vi "MakeExample.vi"(8 "error in (no error)":errorcluster, 9 "TriggerRefractoryPeriod (Frames)":i32, 10 "StimulusObject Parameters":variant, 11 "FullWormGWN in":refnum<class "FullWormGWN.lvclass">) -> (0 "error out":errorcluster, 3 "FullWormGWN out":refnum<class "FullWormGWN.lvclass">)   [LabVIEW 2019, in "FullWormGWN.lvclass"]
uses:
  FullWormGWN.lvclass
  FullWormGWNInputCluster.ctl
  FullWormGWN.lvclass/FullWormGWN.ctl
  ParametersGlobal.vi
  StimulusObject.lvclass
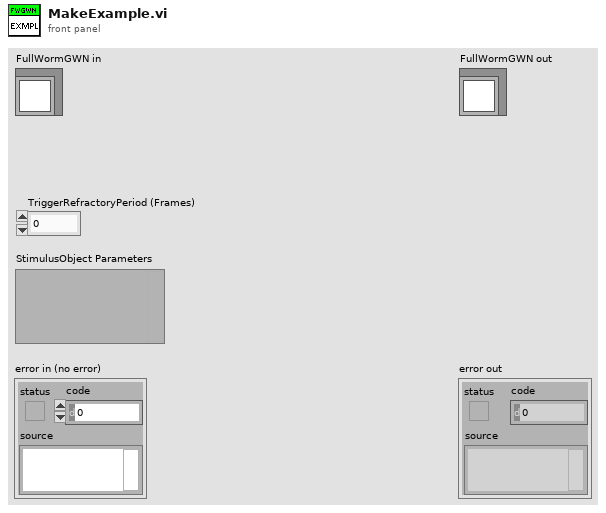
[diagram p1: front panel]
types:
  T1 = typedef "FullWormGWN.lvclass/FullWormGWNInputCluster.ctl" = cluster{"offset (red uW/mm^2m, blue is negative)":sgl, "correlation time (s)":sgl, "standard deviation (red uW/mm^2)":sgl, "Max blue stimulus (uW/mm^2)":sgl, "Max red stimulus (uW/mm^2)":sgl, "dot radius (mm)":sgl}
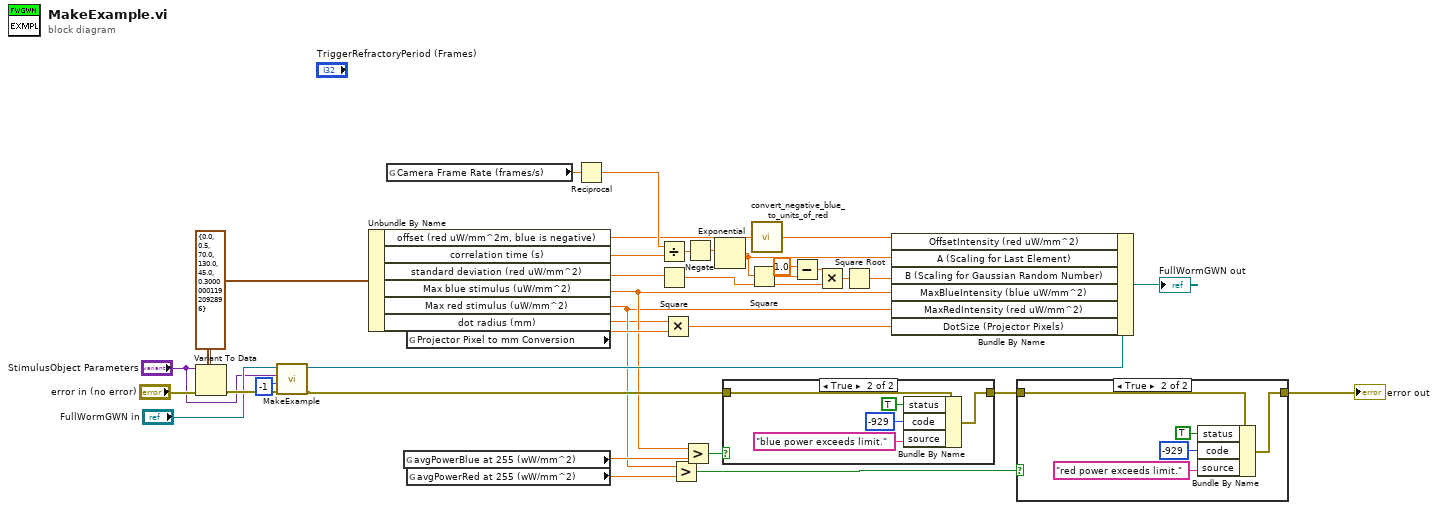
[diagram p0: block diagram]
diagram:
  n1 = Variant To Data(error in="error in (no error)", type=T1 {"offset (red uW/mm^2m, blue is negative)"=0.0, "correlation time (s)"=0.5, "standard deviation (red uW/mm^2)"=70.0, "Max blue stimulus (uW/mm^2)"=130.0, "Max red stimulus (uW/mm^2)"=45.0, "dot radius (mm)"=0.3} ("FullWormGWNInputCluster"), Variant="StimulusObject Parameters") -> (data=w15:T1, error out=w14:errorcluster)
  n2 = call-parent "MakeExample.vi"("error in (no error)"=w14, "TriggerRefractoryPeriod (Frames)"=-1, "StimulusObject Parameters"="StimulusObject Parameters", "StimulusObject in"="FullWormGWN in") -> ("error out"=w20:errorcluster, "StimulusObject out"=w36:refnum<class "FullWormGWN.lvclass">)  [unwired: 6 in]
  n3 = Unbundle By Name(w15) -> ("offset (red uW/mm^2m, blue is negative)"=w7:sgl, "correlation time (s)"=w13:sgl, "standard deviation (red uW/mm^2)"=w12:sgl, "Max blue stimulus (uW/mm^2)"=w11:sgl, "Max red stimulus (uW/mm^2)"=w10:sgl, "dot radius (mm)"=w9:sgl)
  n4 = global read "ParametersGlobal.vi" "Camera Frame Rate (frames/s)"() -> (w27:sgl)
  n5 = global read "ParametersGlobal.vi" "avgPowerBlue at 255 (wW/mm^2)"() -> (w22:sgl)
  n6 = global read "ParametersGlobal.vi" "Projector Pixel to mm Conversion"() -> (w26:sgl)
  n7 = global read "ParametersGlobal.vi" "avgPowerRed at 255 (wW/mm^2)"() -> (w21:sgl)
  n8 = Reciprocal(x=w27) -> (1/x=w29:sgl)
  n9 = Divide(x=w29, y=w13) -> (x/y=w30:sgl)
  n10 = Square(x=w12) -> (x^2=w34:sgl)
  n11 = Multiply(x=w9, y=w26) -> (x*y=w25:sgl)
  n12 = Greater?(x=w10, y=w21) -> (0:w17:bool)
  n13 = Greater?(x=w11, y=w22) -> (0:w19:bool)
  n14 = Negate(x=w30) -> (-x=w31:sgl)
  n15 = Exponential(1:w31) -> (0:w24:sgl)
  n16 = case shown="True" w19 {
    tunnel: w20 -> [w37 w42]
    tunnel: [w37 w41] -> w18
    frame False {
    }
    frame True {
      n17 = Bundle By Name(cluster=w42, "status"=TRUE, "code"=-929, "source"="blue power exceeds limit.") -> (w41:errorcluster)
    }
  }
  n18 = Square(x=w24) -> (x^2=w32:sgl)
  n19 = call "convert_negative_blue_to_units_of_red.vi"("Intensity in units of red (positive) and blue (negative)"=w7) -> ("Intensity in units of red (positive and negative)"=w6:sgl)
  n20 = Subtract(x=sgl 1.0, y=w32) -> (x-y=w33:sgl)
  n21 = Multiply(x=w33, y=w34) -> (x*y=w35:sgl)
  n22 = Square Root(x=w35) -> (sqrt(x)=w23:sgl)
  n23 = Bundle By Name(cluster=w36, "OffsetIntensity (red uW/mm^2)"=w6, "A (Scaling for Last Element)"=w24, "B (Scaling for Gaussian Random Number)"=w23, "MaxBlueIntensity (blue uW/mm^2)"=w11, "MaxRedIntensity (red uW/mm^2)"=w10, "DotSize (Projector Pixels)"=w25) -> (→"FullWormGWN out":refnum<class "FullWormGWN.lvclass">)
  n24 = case shown="True" w17 {
    tunnel: w18 -> [w43 w48]
    tunnel: [w43 w47] -> w1
    frame False {
    }
    frame True {
      n25 = Bundle By Name(cluster=w48, "status"=TRUE, "code"=-929, "source"="red power exceeds limit.") -> (w47:errorcluster)
    }
  }
  "error out" <- w1
